vi "Add Config File Dependency.vi"(8 "error in (no error)":errorcluster, 11 "Item Ref in":T1 format="%.0x") -> (0 "error out":errorcluster, 2 "configuration file set?":bool, 3 "Device Ref out":T1 format="%.0x")   [LabVIEW 2019, in "DSF System Explorer.lvlib"]
uses:
  DSF System Explorer.lvlib
  <vilib>/NI VeriStand/Custom Device API/Custom Device Item Ref.ctl
  <vilib>/NI VeriStand/Custom Device API/Custom Device File Dependency.ctl
  <vilib>/NI VeriStand/Custom Device API/Path Specification.ctl
  <vilib>/NI VeriStand/Custom Device API/Path Type.ctl
  <vilib>/NI VeriStand/Custom Device API/Custom Device Supported Target.ctl
  <vilib>/NI VeriStand/Custom Device API/Get Item Property (Path).vi
  <vilib>/NI VeriStand/Custom Device API/Custom Device API.lvlib
  Shared/DSF Shared.lvlib
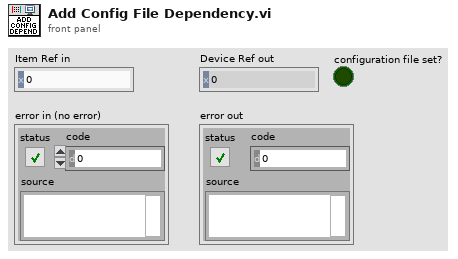
[diagram p1: front panel]
types:
  T1 = typedef "Custom Device API.lvlib/Custom Device Item Ref.ctl" = u64
  T2 = typedef "Custom Device API.lvlib/Custom Device Supported Target.ctl" = enum16{"All", "PharLap", "VxWorks", "Windows", "Linux_32_ARM", "Linux_x64", "PharLap & Windows", "PharLap & VxWorks", "VxWorks & Windows"}
  T3 = typedef "Custom Device API.lvlib/Path Type.ctl" = enum16{"Absolute", "To Base", "To Common Data Dir", "To Application Data Dir"}
  T4 = typedef "Custom Device API.lvlib/Custom Device File Dependency.ctl" = cluster{"Source":T5, "RT Destination":path, "ForceDownload?":bool, "SupportedTarget":T2, "Version":string}
  T5 = typedef "Custom Device API.lvlib/Path Specification.ctl" = cluster{"Path":path, "Type":T3}
  T6 = typedef "Custom Device API.lvlib/Custom Device Target Type.ctl" = enum16{"PharLap", "VxWorks", "Windows", "Linux_32_ARM", "Linux_x64"}
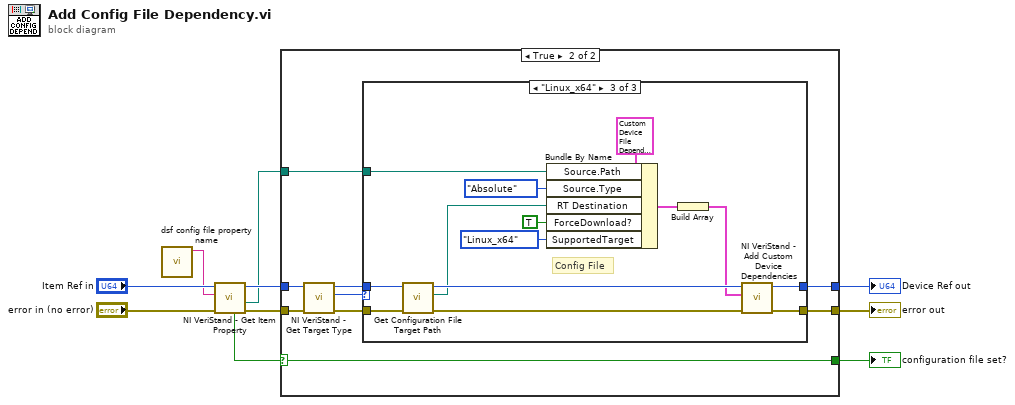
[diagram p0: block diagram]
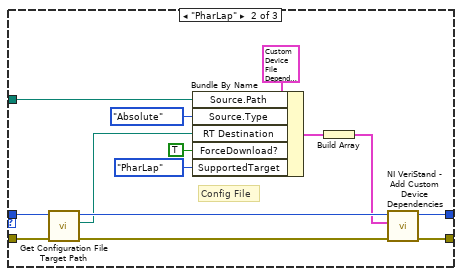
[diagram p4: hidden frame]
diagram:
  n1 = call "dsf config file property name.vi"() -> ("file path property name"=w4:string)  [unwired: 11 in]
  n2 = call-poly <vilib>:"NI VeriStand - Get Item Property.vi"("error in (no error)"="error in (no error)", "Property Name"=w4, "Item Ref in"="Item Ref in") -> ("error out"=w5:errorcluster, "Value"=w3:path, "Item Ref out"=w6:T1, "Found?"=w2:bool)  [unwired: 5 in]
  n3 = case shown="True" w2 {
    selector: w2 -> [w11 w14]
    tunnel: [w13 w19] -> w10
    tunnel: [w12 w18] -> w9
    tunnel: w6 -> [w13 w17]
    tunnel: w5 -> [w12 w16]
    tunnel: w3 -> [_ w15]
    tunnel: [w11 w14] -> w1
    frame False {
    }
    frame True {
      n4 = call <vilib>:"NI VeriStand - Get Target Type.vi"("error in (no error)"=w16, "Item Ref in"=w17) -> ("error out"=w21:errorcluster, "Target Type"=w22:T6, "Item Ref out"=w20:T1)  [unwired: 7 in]
      n5 = case shown="\"Linux_x64\"" w22 {
        tunnel: [w24 w36 w50] -> w18
        tunnel: [w23 w35 w49] -> w19
        tunnel: w20 -> [w23 w38 w52]
        tunnel: w21 -> [w24 w37 w51]
        tunnel: w15 -> [_ w34 w48]
        frame "Windows", Default {
          # "Don't add dependency for Windows or unsupported target type."
        }
        frame "PharLap" {
          # "Config File"
          n6 = call "Get Configuration File Target Path.vi"("error in (no error)"=w37, "Item Ref in"=w38) -> ("error out"=w28:errorcluster, "configuration target path"=w26:path, "Item Ref out"=w27:T1)  [unwired: 7 in]
          n7 = Bundle By Name(cluster=T4 {"Source"={"Path"=path "", "Type"=enum."Absolute"}, "RT Destination"=path "", "ForceDownload?"=FALSE, "SupportedTarget"=enum."PharLap", "Version"=""} ("Dependencies"), "Source.Path"=w34, "Source.Type"=Path_Type."Absolute", "RT Destination"=w26, "ForceDownload?"=TRUE, "SupportedTarget"=Custom_Device_Supported_Target."PharLap") -> (w29:T4)
          n8 = Build Array(w29) -> (w25:T4[])
          n9 = call <vilib>:"NI VeriStand - Add Custom Device Dependencies.vi"("error in (no error)"=w28, "Dependencies"=w25, "Device Ref in"=w27) -> ("error out"=w36:errorcluster, "Device Ref out"=w35:T1)  [unwired: 7 in]
        }
        frame "Linux_x64" {
          # "Config File"
          n10 = call "Get Configuration File Target Path.vi"("error in (no error)"=w51, "Item Ref in"=w52) -> ("error out"=w42:errorcluster, "configuration target path"=w40:path, "Item Ref out"=w41:T1)  [unwired: 7 in]
          n11 = Bundle By Name(cluster=T4 {"Source"={"Path"=path "", "Type"=enum."Absolute"}, "RT Destination"=path "", "ForceDownload?"=FALSE, "SupportedTarget"=enum."PharLap", "Version"=""} ("Dependencies"), "Source.Path"=w48, "Source.Type"=Path_Type."Absolute", "RT Destination"=w40, "ForceDownload?"=TRUE, "SupportedTarget"=Custom_Device_Supported_Target."Linux_x64") -> (w43:T4)
          n12 = Build Array(w43) -> (w39:T4[])
          n13 = call <vilib>:"NI VeriStand - Add Custom Device Dependencies.vi"("error in (no error)"=w42, "Dependencies"=w39, "Device Ref in"=w41) -> ("error out"=w50:errorcluster, "Device Ref out"=w49:T1)  [unwired: 7 in]
        }
      }
    }
  }
  "Device Ref out" <- w10
  "error out" <- w9
  "configuration file set?" <- w1
